vi "SubVI_SVM_Confusion_Matrix.vi"(10 "Real Labels":dbl[][](array[numeric]), 11 "Predictions":dbl[][](array[numeric])) -> (9 "Performance":T1)   [LabVIEW 2020]
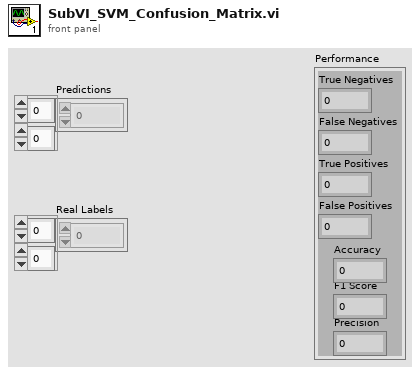
[diagram p1: front panel]
types:
  T1 = cluster{"True Negatives":i32, "False Negatives":i32, "True Positives":i32, "False Positives":i32, "Accuracy":dbl, "F1 Score":dbl, "Precision":dbl}
  T2 = cluster{"True Negatives":i32, "False Negatives":i32, "True Positives":i32, "False Positives":i32, dbl, dbl, dbl}
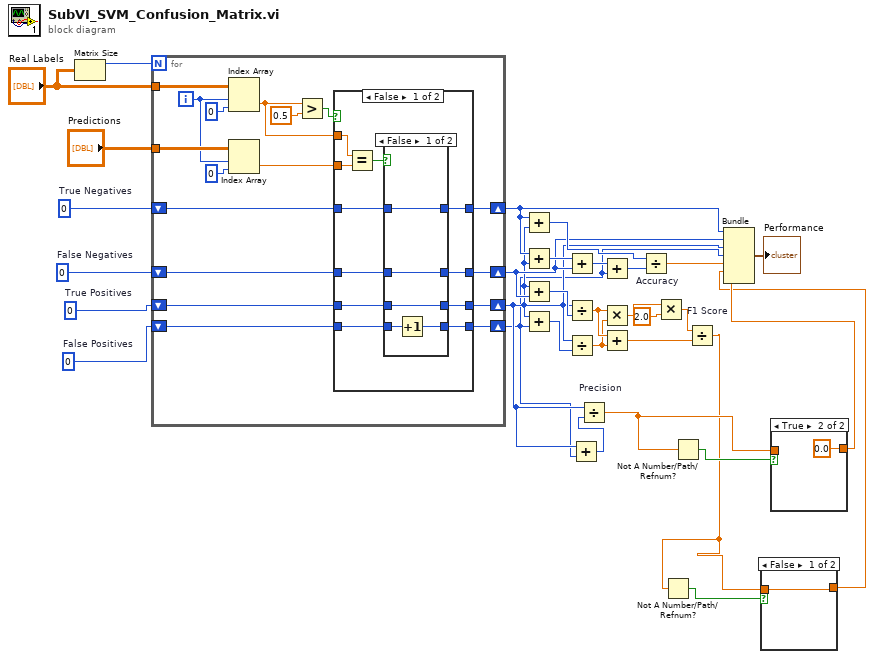
[diagram p0: block diagram]
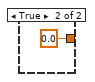
[diagram p2: hidden frame]
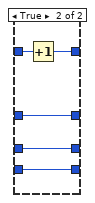
[diagram p4: hidden frame]
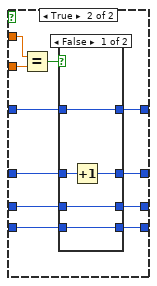
[diagram p5: hidden frame]
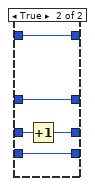
[diagram p6: hidden frame]
diagram:
  w17 = 0  # False Positives
  w16 = 0  # False Negatives
  w14 = 0  # True Negatives
  w15 = 0  # True Positives
  n1 = Matrix Size(0:"Real Labels") -> (1:w18:i32)  [unwired: 1 out]
  n2 = for {
    N: w18 -> [_]
    shift-right: [w48] -> w13
    shift-left: w14 -> [w49]
    shift-right: [w46] -> w10
    shift-left: w15 -> [w47]
    shift-right: [w44] -> w12
    shift-left: w16 -> [w45]
    shift-right: [w42] -> w9
    shift-left: w17 -> [w43]
    tunnel: "Real Labels" -> [w41]
    tunnel: "Predictions" -> [w38]
    i -> [w37]
    n3 = Index Array(array=w41, index (row)=w37, index (col)=0 ("disabled index (col)")) -> (element=w34:dbl)
    n4 = Index Array(array=w38, index (row)=w37, index (col)=0 ("disabled index (col)")) -> (element=w33:dbl)
    n5 = Greater?(x=w34, y=0.5) -> (0:w35:bool)
    n6 = case shown="False" w35 {
      tunnel: w49 -> [w57 w81]
      tunnel: [w56 w80] -> w48
      tunnel: w47 -> [w55 w79]
      tunnel: [w54 w78] -> w46
      tunnel: w45 -> [w53 w77]
      tunnel: [w52 w76] -> w44
      tunnel: w43 -> [w51 w75]
      tunnel: [w50 w74] -> w42
      tunnel: w34 -> [w60 w73]
      tunnel: w33 -> [w59 w72]
      frame False {
        n7 = Equal?(x=w60, y=w59) -> (x = y?=w58:bool)
        n8 = case shown="False" w58 {
          tunnel: w57 -> [w62 w70]
          tunnel: [w62 w66] -> w56
          tunnel: w55 -> [w63 w69]
          tunnel: [w63 w69] -> w54
          tunnel: w53 -> [w64 w68]
          tunnel: [w64 w68] -> w52
          tunnel: w51 -> [w65 w67]
          tunnel: [w61 w67] -> w50
          frame False {
            n9 = Increment(x=w65) -> (x+1=w61:i32)
          }
          frame True {
            n10 = Increment(x=w70) -> (x+1=w66:i32)
          }
        }
      }
      frame True {
        n11 = Equal?(x=w73, y=w72) -> (x = y?=w71:bool)
        n12 = case shown="False" w71 {
          tunnel: w81 -> [w83 w91]
          tunnel: [w83 w91] -> w80
          tunnel: [w84 w87] -> w78
          tunnel: w79 -> [w84 w90]
          tunnel: w77 -> [w85 w89]
          tunnel: [w82 w89] -> w76
          tunnel: w75 -> [w86 w88]
          tunnel: [w86 w88] -> w74
          frame False {
            n13 = Increment(x=w85) -> (x+1=w82:i32)
          }
          frame True {
            n14 = Increment(x=w90) -> (x+1=w87:i32)
          }
        }
      }
    }
  }
  n15 = Add(x=w13, y=w10) -> (x+y=w24:i32)
  n16 = Add(x=w13, y=w10) -> (x+y=w21:i32)
  n17 = Add(x=w10, y=w12) -> (x+y=w25:i32)
  n18 = Add(x=w10, y=w9) -> (x+y=w26:i32)
  n19 = Add(x=w21, y=w12) -> (x+y=w22:i32)
  n20 = Divide(x=w10, y=w25) -> (x/y=w30:dbl)
  n21 = Divide(x=w10, y=w26) -> (x/y=w29:dbl)
  n22 = Add(x=w10, y=w9) -> (x+y=w8:i32)
  n23 = Divide "Precision"(x=w10, y=w8) -> (x/y=w5:dbl)
  n24 = Add(x=w22, y=w9) -> (x+y=w23:i32)
  n25 = Multiply(x=w30, y=w29) -> (x*y=w27:dbl)
  n26 = Add(x=w30, y=w29) -> (x+y=w32:dbl)
  n27 = Divide "Accuracy"(x=w24, y=w23) -> (x/y=w11:dbl)
  n28 = Multiply(x=w27, y=2.0) -> (x*y=w31:dbl)
  n29 = Not A Number/Path/Refnum?(number/path/refnum=w5) -> (NaN/Path/Refnum?=w6:bool)
  n30 = Divide "F1 Score"(x=w31, y=w32) -> (x/y=w2:dbl)
  n31 = Not A Number/Path/Refnum?(number/path/refnum=w2) -> (NaN/Path/Refnum?=w3:bool)
  n32 = case shown="False" w3 {
    tunnel: w2 -> [w92 _]
    tunnel: [w92 0.0] -> w1
    frame False {
    }
    frame True {
    }
  }
  n33 = case shown="True" w6 {
    tunnel: w5 -> [w94 _]
    tunnel: [w94 0.0] -> w4
    frame False {
    }
    frame True {
    }
  }
  n34 = Bundle("True Negatives"=w13, "False Negatives"=w12, "True Positives"=w10, "False Positives"=w9, w11, w1, w4) -> (→"Performance":T2)  [unwired: 1 in]
